vi "Login_Main .vi"() -> ()   [LabVIEW 2022 SP3]
doc: "The application should not allow the user to enter an invalid username and password.\nThe user should be able to log in with valid credentials."
uses:
  1c1b4bb6-12af-42db-9b54-20e657ab4828.vi
  949bb38c-e2e6-4362-8248-b9fc3bdc1f0f.vi
  <vilib>/Utility/error.llb/Trim Whitespace One-Sided.vi
  <vilib>/Utility/file.llb/Read Delimited Spreadsheet (string).vi
  <vilib>/Utility/file.llb/Write Delimited Spreadsheet (string).vi
panel:
  in  "error in":errorcluster
  in  "Enter":bool
  in  "Stop Button":bool
  out "Pass = True":bool
  in  "Change Password":bool
  in  "Show Password":bool
  in  "PASSWORD":string
  in  "SELECT USER":i32(ring) items=["Vigneshwaran", "Kannan", "Kamala", "Arul", "Saravanan", "Ajai", "Sarfaraz", "Lingesh"]
  # "Agnikul Cosmos"
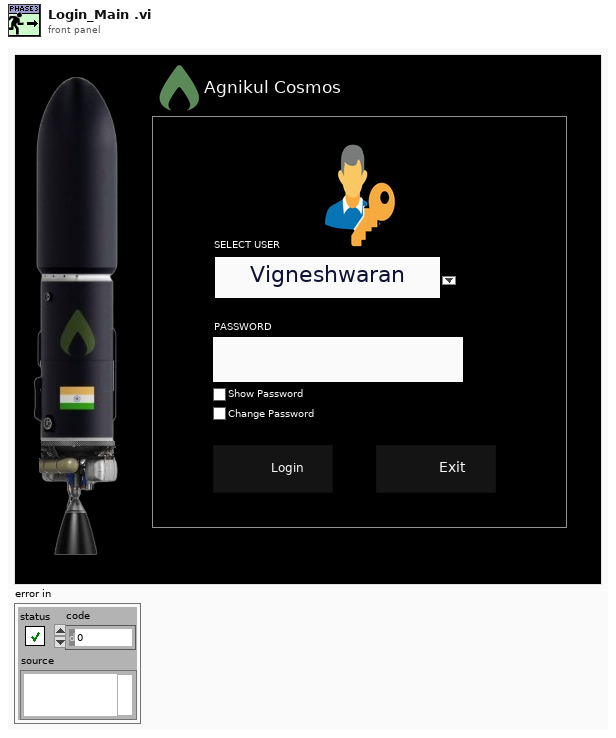
[diagram p1: front panel]
types:
  T1 = cluster{"Datalog path":path, "Configuration path":path, "Signal list path":path, "Sub vi's":path, "Authentication":path}
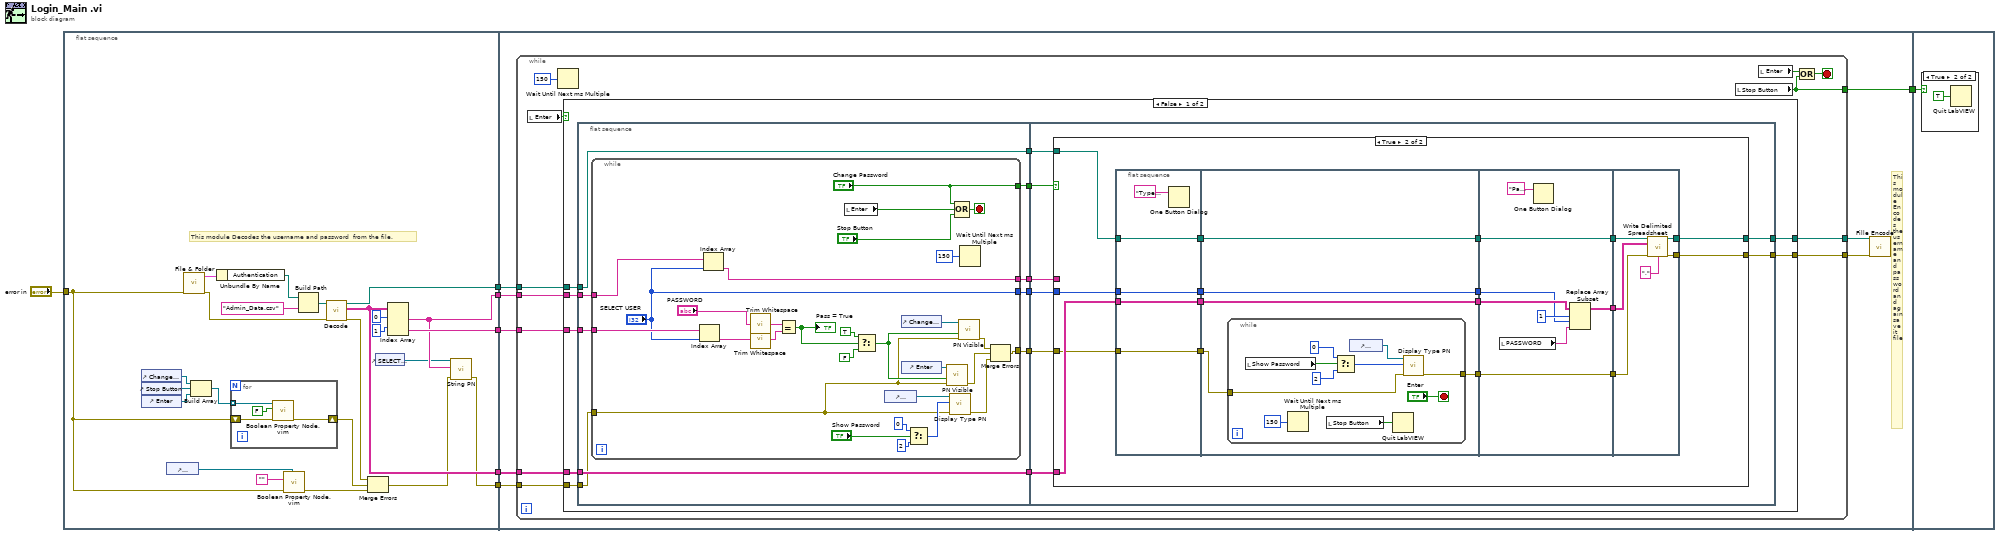
[diagram p0: block diagram]
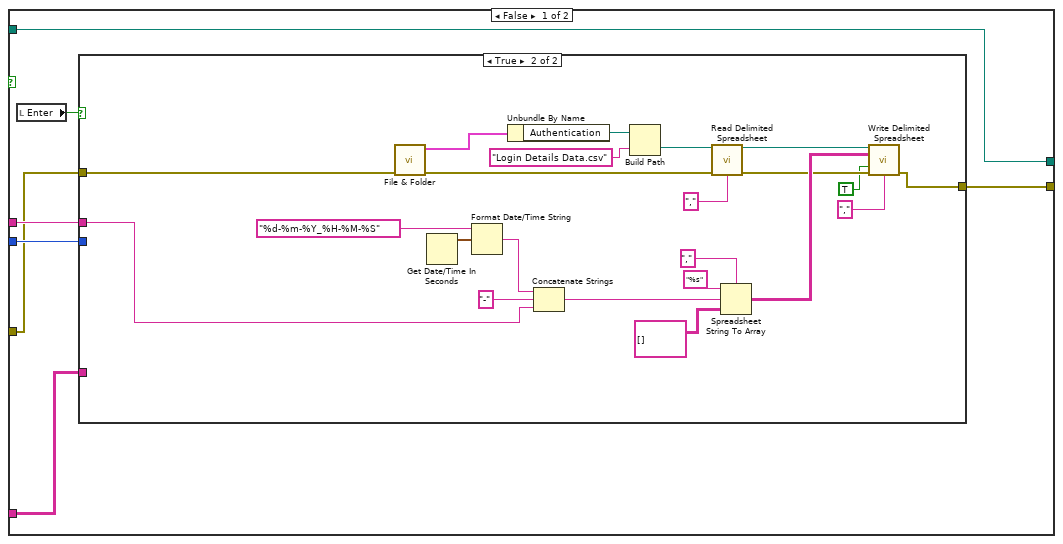
[diagram p2: hidden frame]
diagram:
  n1 = flat-sequence {
    tunnel: [w29] -> w7
    tunnel: [w23] -> w6
    tunnel: [w24] -> w5
    tunnel: [w8] -> w4
    tunnel: [w11] -> w3
    tunnel: "error in" -> [w12]
    tunnel: w4 -> [w36]
    tunnel: w5 -> [w41]
    tunnel: w6 -> [w42]
    tunnel: w7 -> [w43]
    tunnel: w3 -> [w40]
    tunnel: [w39] -> w2
    tunnel: w2 -> [w198]
    frame #0 {
      # "This module Decodes the username and password  from the file."
      n2 = control-ref of="Change Password"() -> (w18:refnum<vi>)
      n3 = control-ref of="Stop Button"() -> (w19:refnum<vi>)
      n4 = control-ref of="Enter"() -> (w20:refnum<vi>)
      n5 = control-ref of="PASSWORD"() -> (w16:refnum<vi>)
      n6 = call "File & Folder.vi"("error in (no error)"=w12) -> ("error out"=w22:errorcluster, "Cluster"=w27:T1)  [unwired: 9 in]
      n7 = Build Array(w18, w19, w20) -> (w17:refnum<vi>[])
      n8 = Unbundle By Name(w27) -> ("Authentication"=w26:path)
      n9 = for {
        tunnel: w17 -> [w35] mode=indexing
        shift-right: [w32] -> w13
        shift-left: w12 -> [w33]
        n10 = call "Boolean Property Node.vim"("error in (no error)"=w33, "String"=FALSE ("Value"), "Boolean 2"=w35) -> ("error out"=w32:errorcluster)  [unwired: 5 in, 3 out]
      }
      n11 = call "Boolean Property Node.vim"("String 2"=w16, "error in (no error)"=w12, "String"="" ("Empty String Constant")) -> ("error out"=w14:errorcluster)  [unwired: 5 in, 3 out]
      n12 = Build Path(base path=w26, name or relative path="Admin_Data.csv" ("name")) -> (appended path=w25:path)
      n13 = call "Decode.vi"("error IO"=w22, "Encoded  File"=w25) -> ("error out"=w21:errorcluster, "Decoded Value"=w23:string[][], "Decoded File"=w24:path)  [unwired: 7 in]
      n14 = Merge Errors(w21, w13, w14) -> (w9:errorcluster)
      n15 = control-ref of="SELECT USER"() -> (w10:refnum<vi>)
      n16 = Index Array(array=w23, index (row) #1=0 ("index (row)"), index (row) #2=1 ("index (row)")) -> (element #1=w11:string[], element #2=w29:string[])  [unwired: 2 in]
      n17 = call "String PN.vi"("error in (no error)"=w9, "Strings []"=w11, "reference"=w10) -> ("error out"=w8:errorcluster)  [unwired: 7 in, 1 out]
    }
    frame #1 {
      # "This module Encodes the username and password and  again  save it file"
      n18 = while {
        tunnel: w43 -> [w54]
        tunnel: w42 -> [w53]
        tunnel: w41 -> [w52]
        tunnel: w40 -> [w50]
        tunnel: [w47] -> w39
        tunnel: [w46] -> w37
        tunnel: [w45] -> w38
        tunnel: w36 -> [w44]
        stop <- w49 stop-if-true
        n19 = local read "Enter"() -> (w51:bool)
        n20 = Wait Until Next ms Multiple(millisecond multiple=u32 150) -> ()  [unwired: 1 out]
        n21 = case shown="False" w51 {
          tunnel: w54 -> [w66 _]
          tunnel: w53 -> [w65 _]
          tunnel: w52 -> [w62 w197]
          tunnel: w50 -> [w61 _]
          tunnel: [w60 w196] -> w46
          tunnel: [w59 w197] -> w45
          tunnel: w44 -> [w57 w196]
          frame False {
            n22 = flat-sequence {
              tunnel: [w77] -> w68
              tunnel: [w76] -> w67
              tunnel: [w74] -> w64
              tunnel: [w71] -> w63
              tunnel: [w72] -> w58
              tunnel: w65 -> [w77]
              tunnel: w66 -> [w75]
              tunnel: w62 -> [w71]
              tunnel: w61 -> [w73]
              tunnel: w57 -> [w70]
              tunnel: [w69] -> w56
              tunnel: w68 -> [w114]
              tunnel: w67 -> [w113]
              tunnel: w64 -> [w112]
              tunnel: w63 -> [w109]
              tunnel: [w111] -> w59
              tunnel: [w110] -> w60
              tunnel: w58 -> [w108]
              tunnel: w56 -> [w107]
              frame #0 {
                n23 = while {
                  tunnel: ["SELECT USER"] -> w76
                  tunnel: w75 -> [w106]
                  tunnel: ["Change Password"] -> w74
                  tunnel: w73 -> [w95]
                  tunnel: [w94] -> w72
                  tunnel: w70 -> [w79]
                  tunnel: [w80] -> w69
                  stop <- w99 stop-if-true
                  n24 = Index Array(array=w106, index="SELECT USER") -> (element=w105:string)
                  n25 = Index Array(array=w95, index="SELECT USER") -> (element=w94:string)
                  n26 = call <vilib>:"Trim Whitespace.vi"("string"="PASSWORD") -> ("trimmed string"=w101:string)  [unwired: 1 in]
                  n27 = call <vilib>:"Trim Whitespace.vi"("string"=w105) -> ("trimmed string"=w96:string)  [unwired: 1 in]
                  n28 = Equal?(x=w101, y=w96) -> (x = y?=w90:bool)
                  "Pass = True" <- w90
                  n29 = local read "Enter"() -> (w97:bool)
                  n30 = Select(t=TRUE, s=w90, f=FALSE ("Visible")) -> (s? t:f=w91:bool)
                  n31 = control-ref of="PASSWORD"() -> (w86:refnum<vi>)
                  n32 = control-ref of="Change Password"() -> (w93:refnum<vi>)
                  n33 = control-ref of="Enter"() -> (w92:refnum<vi>)
                  n34 = Select(t=u32 0 ("Display Style"), s="Show Password", f=u32 2 ("Display Style")) -> (s? t:f=w85:u32)
                  n35 = call "PN Visible.vi"("error in"=w79, "Visible"=w91, "reference"=w92) -> ("error out"=w81:errorcluster)  [unwired: 8 in]
                  n36 = call "Display Type PN.vi"("error in"=w79, "s? t:f"=w85, "reference"=w86) -> ("error out"=w78:errorcluster)  [unwired: 7 in, 1 out]
                  n37 = Compound Arithmetic op=OR("Change Password", w97, "Stop Button") -> (w99:bool)
                  n38 = call "PN Visible.vi"("error in"=w79, "Visible"=w91, "reference"=w93) -> ("error out"=w82:errorcluster)  [unwired: 8 in]
                  n39 = Wait Until Next ms Multiple(millisecond multiple=u32 150) -> ()  [unwired: 1 out]
                  n40 = Merge Errors(w82, w81, w78) -> (w80:errorcluster)
                }
              }
              frame #1 {
                n41 = case shown="True" w112 {
                  tunnel: w114 -> [w121 w159]
                  tunnel: w113 -> [w120 w156]
                  tunnel: w109 -> [w118 w151]
                  tunnel: [w118 w150] -> w111
                  tunnel: [w115 w149] -> w110
                  tunnel: w108 -> [w117 _]
                  tunnel: w107 -> [w116 w148]
                  frame False {
                    n42 = local read "Enter"() -> (w119:bool)
                    n43 = case shown="True" w119 {
                      tunnel: w121 -> [_ _]
                      tunnel: w120 -> [_ _]
                      tunnel: w117 -> [_ w142]
                      tunnel: w116 -> [w122 w141]
                      tunnel: [w122 w139] -> w115
                      frame False {
                      }
                      frame True {
                        n44 = call "File & Folder.vi"("error in (no error)"=w141) -> ("error out"=w125:errorcluster, "Cluster"=w136:T1)  [unwired: 9 in]
                        n45 = Get Date/Time In Seconds() -> (seconds since 1Jan1904=w132:timestamp)
                        n46 = Format Date/Time String(time format string (%c)="%d-%m-%Y_%H-%M-%S", seconds (now)=w132) -> (date/time string=w127:string)  [unwired: 1 in]
                        n47 = Unbundle By Name(w136) -> ("Authentication"=w135:path)
                        n48 = Concatenate Strings(w127, "-" ("string"), w142) -> (w128:string)
                        n49 = Build Path(base path=w135, name or relative path="Login Details Data.csv" ("name")) -> (appended path=w134:path)
                        n50 = call-poly <vilib>:"Read Delimited Spreadsheet.vi"("file path (dialog if empty)"=w134, "error in (no error)"=w125, "delimiter (\\t)"="," ("delimiter (\\t)")) -> ("new file path (Not A Path if cancelled)"=w144:path, "error out"=w140:errorcluster)  [unwired: 7 in, 4 out]
                        n51 = Spreadsheet String To Array(delimiter (Tab)=",", format string="%s", spreadsheet string=w128, array type (2D Dbl)=string[][] [] ("all rows")) -> (array=w143:string[][])
                        n52 = call-poly <vilib>:"Write Delimited Spreadsheet.vi"("file path (dialog if empty)"=w144, "2D data"=w143, "append to file? (new file:F)"=TRUE, "error in (no error)"=w140, "delimiter (\\t)"="," ("delimiter (\\t)")) -> ("error out"=w139:errorcluster)  [unwired: 9 in, 1 out]
                      }
                    }
                  }
                  frame True {
                    n53 = flat-sequence {
                      tunnel: [w166] -> w160
                      tunnel: w159 -> [w166]
                      tunnel: [w165] -> w157
                      tunnel: w156 -> [w165]
                      tunnel: [w164] -> w152
                      tunnel: w151 -> [w164]
                      tunnel: w148 -> [w162]
                      tunnel: [w162] -> w147
                      tunnel: [w171] -> w161
                      tunnel: w160 -> [w171]
                      tunnel: [w170] -> w158
                      tunnel: w157 -> [w170]
                      tunnel: [w169] -> w153
                      tunnel: w152 -> [w169]
                      tunnel: w147 -> [w168]
                      tunnel: [w167] -> w145
                      tunnel: w161 -> [w188]
                      tunnel: w158 -> [w182]
                      tunnel: [w185] -> w155
                      tunnel: [w184] -> w154
                      tunnel: w153 -> [w184]
                      tunnel: [w183] -> w146
                      tunnel: w145 -> [w183]
                      tunnel: w155 -> [w195]
                      tunnel: w154 -> [w194]
                      tunnel: [w192] -> w150
                      tunnel: [w191] -> w149
                      tunnel: w146 -> [w190]
                      frame #0 {
                        n54 = One Button Dialog(message="Type New Password and Press Enter button") -> ()  [unwired: 1 in, 1 out]
                      }
                      frame #1 {
                        n55 = while {
                          tunnel: w168 -> [w173]
                          tunnel: [w172] -> w167
                          stop <- "Enter" stop-if-true
                          n56 = local read "Show Password"() -> (w176:bool)
                          n57 = Wait Until Next ms Multiple(millisecond multiple=u32 150) -> ()  [unwired: 1 out]
                          n58 = local read "Stop Button"() -> (w180:bool)
                          n59 = Select(t=u32 0 ("Display Style"), s=w176, f=u32 2 ("Display Style")) -> (s? t:f=w174:u32)
                          n60 = control-ref of="PASSWORD"() -> (w175:refnum<vi>)
                          n61 = Quit LabVIEW(quit? (T)=w180) -> ()
                          n62 = call "Display Type PN.vi"("error in"=w173, "s? t:f"=w174, "reference"=w175) -> ("error out"=w172:errorcluster)  [unwired: 7 in, 1 out]
                        }
                      }
                      frame #2 {
                        n63 = local read "PASSWORD"() -> (w186:string)
                        n64 = One Button Dialog(message="Password changed successfully, Please Login with new Password") -> ()  [unwired: 1 in, 1 out]
                        n65 = Replace Array Subset(array=w188, new element=w186, index (row)=1, index (col)=w182) -> (w185:string[][])
                      }
                      frame #3 {
                        n66 = call-poly <vilib>:"Write Delimited Spreadsheet.vi"("file path (dialog if empty)"=w194, "2D data"=w195, "error in (no error)"=w190, "delimiter (\\t)"="," ("delimiter (\\t)")) -> ("new file path (Not A Path if cancelled)"=w192:path, "error out"=w191:errorcluster)  [unwired: 10 in]
                      }
                    }
                  }
                }
              }
            }
          }
          frame True {
          }
        }
        n67 = local read "Stop Button"() -> (w47:bool)
        n68 = local read "Enter"() -> (w48:bool)
        n69 = Compound Arithmetic op=OR(w48, w47) -> (w49:bool)
      }
      n70 = call "Fille Encode.vi"("error in"=w37, "Original File"=w38) -> ()  [unwired: 8 in, 2 out]
    }
    frame #2 {
      n71 = case shown="True" w198 {
        frame False {
        }
        frame True {
          n72 = Quit LabVIEW(quit? (T)=TRUE) -> ()
        }
      }
    }
  }
